vi "Ground Station to Aircraft Coms Main.vi"(11 "Instance Details":T16) -> ()   [LabVIEW 2014]
uses:
  Application Support/Stop Button/SubVI/Get Stop Button Status.vi
  MAVLink/Commands/MAV_CMD Sub VI/MAV_CMD_COMPONENT_ARM_DISARM.vi
  Telemetry/Controls/Aircraft State.ctl
  Aircraft Information/Sub VI/Get Aircraft System Status.vi
  Aircraft Information/Sub VI/Set Aircraft System Status.vi
  Aircraft Information/Sub VI/Get Aircraft Attitude.vi
  Aircraft Information/Sub VI/Get Aircraft RC.vi
  Aircraft Information/Sub VI/Get Aircraft Information.vi
  Aircraft Information/Sub VI/Get Aircraft Extra Data.vi
  Aircraft Information/Sub VI/Get Aircraft GPS.vi
  Aircraft Information/Controls/Aircraft RC Data.ctl
  Aircraft Information/Controls/Aircraft Attitude Data.ctl
  Aircraft Information/Controls/Base Mode.ctl
  Aircraft Information/Controls/Drone Information.ctl
  Aircraft Information/Controls/Aircraft Mode.ctl
  Aircraft Information/Controls/Aircraft Sensor Status Data.ctl
  GUI Design/Indicators/Status LED.ctl
  GUI Design/Indicators/Sensor Status LED CLuster.ctl
  Telemetry/Controls/Telemetry Connection Type.ctl
  SubVI/Aircraft Data Router/Controls/Known Aircraft.ctl
  SubVI/Hardware Driver/Controls/Coms Driver Interface.ctl
  MAVLink/Controls/MAVLink Optical Flow.ctl
  MAVLink/Controls/MAVLink EKF Status Report.ctl
  Aircraft Information/Controls/Aircraft Extra Data.ctl
  Aircraft Information/Controls/Aircraft GPS Data.ctl
  <vilib>/httpClient/ClientHandle.ctl
  <vilib>/httpClient/LabVIEWHTTPClient.lvlib
  Aircraft Information/Controls/GPS Fix Type.ctl
panel:
  in  "Aircraft State":T1=enum."Initialise"
  in  "Main Tab":T2(tab)
  out "Drone Information":T3={"Aircraft ID"=0, "Tag ID"="", "System Status"="", "Base Mode"={"Custom Mode"=FALSE, "Test Enabled"=FALSE, "Autonomous Mode"=FALSE, "Guided Mode"=FALSE, "Stabilization Enabled"=FALSE, "HIL Enabled"=FALSE, "Manual Mode"=FALSE, "Arm"=FALSE}, "Armed/Disarmed"=FALSE, "Battery Voltage"=0.0, "Control Mode"=enum."Stabalise", "Initialisation"=0, "Coms with aircraft good"=FALSE, "Mode"="", "Mission Uploaded"=FALSE} {"Initialisation" scale=0.0..100.0}
  out "Aircraft GPS Data Out":T6
  in  "ARM/DISARM":bool
  in  "Takeoff":bool
  in  "Altitude (m)":sgl
  out "Aircraft Att Data Out":T8
  out "System Status Out":T9 {"Communication Drop Rate (%)" scale=0.0..100.0; "Battery Remaining (%)" scale=0.0..100.0; "CPU Load (%)" scale=0.0..100.0}
  out "Status text":string
  in  "Clear Status Text":bool
  out "Extra Data Out":T12
  out "TX Queue State":i32(slide) scale=0.0..50.0
  out "RX Queue State":i32(slide) scale=0.0..50.0
  out "Waypoint Queue State":i32(slide) scale=0.0..50.0
  in  "param_id":string
  in  "Request Param":bool
  in  "Get Message":bool
  in  "Message Rate (hz)":u16=5
  in  "start_stop":bool
  in  "req_stream_id":T15(ring)
  in  "Release Control":bool
  out "Aircraft RC Data Out":T20
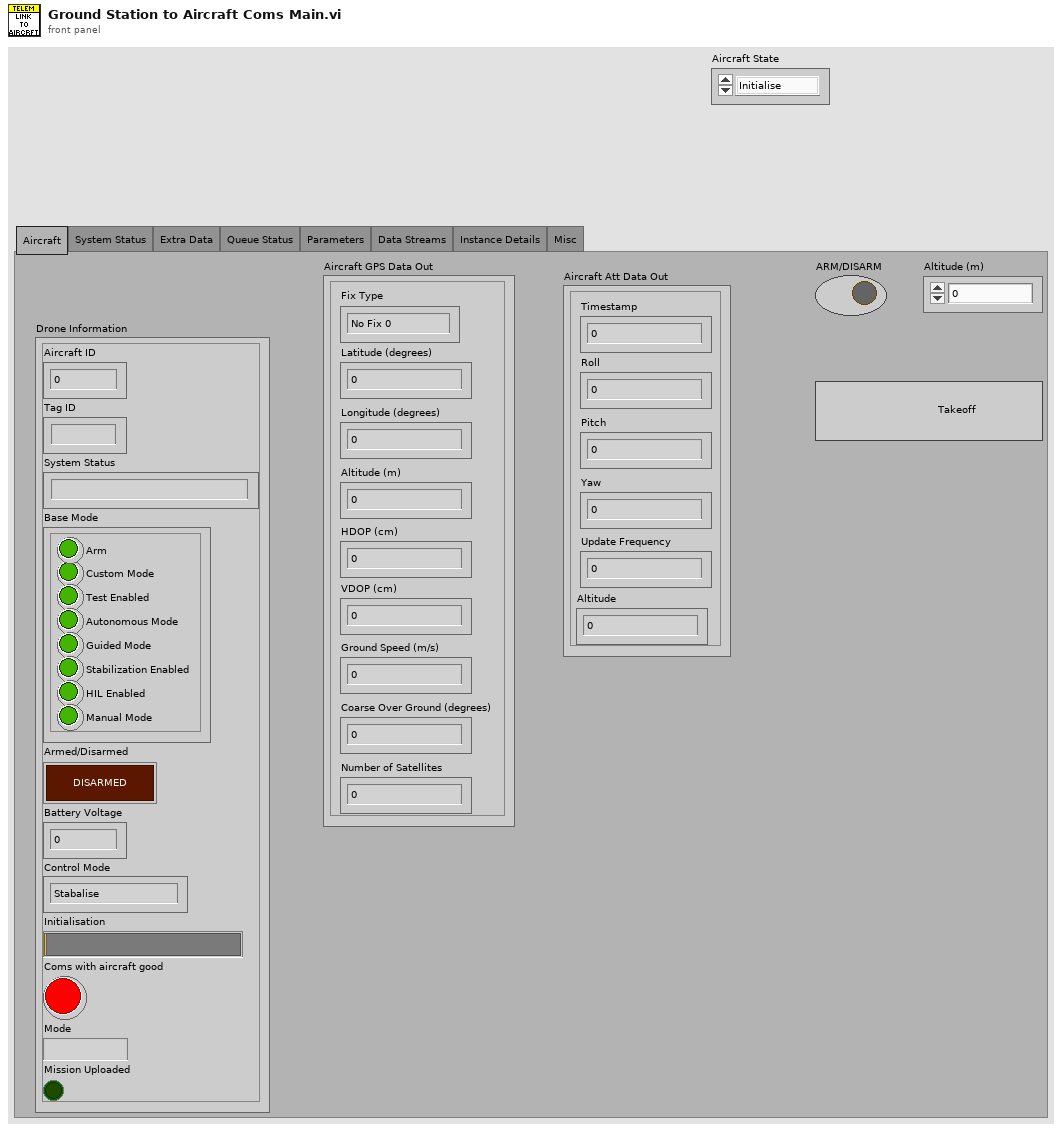
[diagram p1: front panel]
types:
  T1 = typedef "Aircraft State.ctl" = enum16{"Connected", "Initialise", "Disconnected"}
  T2 = enum32{"Aircraft", "System Status", "Extra Data", "Queue Status", "Parameters", "Data Streams", "Instance Details", "Misc"}
  T3 = typedef "Drone Information.ctl" = cluster{"Aircraft ID":u8, "Tag ID":string, "System Status":string, "Base Mode":T4, "Armed/Disarmed":bool, "Battery Voltage":dbl, "Control Mode":T5, "Initialisation":u8, "Coms with aircraft good":bool, "Mode":string, "Mission Uploaded":bool}
  T4 = typedef "Base Mode.ctl" = cluster{"Custom Mode":bool, "Test Enabled":bool, "Autonomous Mode":bool, "Guided Mode":bool, "Stabilization Enabled":bool, "HIL Enabled":bool, "Manual Mode":bool, "Arm":bool}
  T5 = typedef "Aircraft Mode.ctl" = enum16{"Loiter", "Stabalise", "Failsafe", "Emergency Stop"}
  T6 = typedef "Aircraft GPS Data.ctl" = cluster{"Latitude (degrees)":dbl, "Longitude (degrees)":dbl, "Altitude (m)":dbl, "Fix Type":T7, "HDOP (cm)":u16, "VDOP (cm)":u16, "Ground Speed (m/s)":dbl, "Coarse Over Ground (degrees)":u16, "Number of Satellites":u8}
  T7 = typedef "GPS Fix Type.ctl" = enum16{"No Fix 0", "No Fix 1", "2D Fix", "3D Fix", "DGPS", "RTK"}
  T8 = typedef "Aircraft Attitude Data.ctl" = cluster{"Roll":sgl, "Pitch":sgl, "Yaw":sgl, "Timestamp":u32, "Update Frequency":dbl, "Altitude":sgl}
  T9 = typedef "Aircraft Sensor Status Data.ctl" = cluster{"Sensor Status":T10, "CPU Load (%)":dbl, "Battery Voltage (V)":dbl, "Battery Current (A)":dbl, "Battery Remaining (%)":dbl, "Communication Drop Rate (%)":dbl, "Communication Errors (%)":dbl, "Status text":string}
  T10 = typedef "Sensor Status LED CLuster.ctl" = cluster{"3D Gyro":u32, "3D Accel":u32, "3D Mag":u32, "Abs. Pressure":u32, "Diff. Pressure":u32, "GPS":T11, "Optical Flow":u32, "Vision Position":u32, "Laser Position":u32, "External Ground Truth":u32, "Angular Rate Control":u32, "Attitude Stabilisation":u32, "Yaw Position":u32, "Z Altitude Control":u32, "XY Position Control":u32, "Motor Outputs":u32, "RC Receiver":u32, "3D Gyro 2":u32, "3D Accel 2":u32, "3D Mag 2":u32, "Geofence":u32, "AHRS":u32, "Terrain":u32}
  T11 = typedef "Status LED.ctl" = u32
  T12 = typedef "Aircraft Extra Data.ctl" = cluster{"Optical Flow":T13, "RNGFND Distance (m)":sgl, "RNGFND Voltage":sgl, "EKF Status Report":T14}
  T13 = typedef "MAVLink Optical Flow.ctl" = cluster{"Time (usec)":u64, "Flow Comp mx":sgl, "Flow Comp my":sgl, "Ground Distance (m)":sgl, "Flow x":i16, "Flow y":i16, "Sensord ID":u8, "Quality":u8}
  T14 = typedef "MAVLink EKF Status Report.ctl" = cluster{"EKF Status Flags":cluster{"Attitude Estimate":bool, "Horizontal Velocity":bool, "Vertical Velocity":bool, "Horizontal POS Relative":bool, "Horizontal POS Absolute":bool, "Vertical POS Relative":bool, "Vertical POS Absolute":bool, "Vertical POS AGL":bool, "Contstant POS Mode":bool, "Predicted Horizontal POS Relative":bool, "Predicted Horizontal POS Absolute":bool}, "Velocity Variance":sgl, "Horizontal POS Variance":sgl, "Vertical POS Variance":sgl, "Compass Variance":sgl, "Terrain Altitude Variance":sgl}
  T15 = enum16{"ALL", "RAW_SENSORS", "EXTENDED_STATUS", "RC_CHANNELS", "RAW_CONTROLLER", "POSITION", "EXTRA1", "EXTRA2", "EXTRA3"}
  T16 = typedef "Known Aircraft.ctl" = cluster{"Aircraft ID":u8, "Aircraft Receive queue Ref":refnum<queue>, "Aircraft Transmit queue Ref":refnum<queue>, "Waypoint Queue Ref":refnum<queue>, "Connection Details":T17}
  T17 = typedef "Coms Driver Interface.ctl" = cluster{"Connection Type":T18, "UDP connection ID":refnum<k16>, "Serial COM port ID":refnum<visa-resource-name>, "IP Address of Aircraft":u32, "Remote Master Details":cluster{"Remote Master client handle":T19, "Base Path of Web Service":string}, "UDP TX Port of Aircraft":u16}
  T18 = typedef "Telemetry Connection Type.ctl" = enum16{"Serial", "UDP", "Remote Master"}
  T19 = typedef "LabVIEWHTTPClient.lvlib/ClientHandle.ctl" = refnum<k1>
  T20 = typedef "Aircraft RC Data.ctl" = cluster{"Channel 1 Min":i16, "Channel 1 Max":i16, "Channel 2 Min":i16, "Channel 2 Max":i16, "Channel 3 Min":i16, "Channel 3 Max":i16, "Channel 4 Min":i16, "Channel 4 Max":i16}
  T21 = cluster{"req_message_rate":u16, "target_system":u8, "target_component":u8, "req_stream_id":enum16{"ALL", "RAW_SENSORS", "EXTENDED_STATUS", "RC_CHANNELS", "RAW_CONTROLLER", "POSITION", "EXTRA1", "EXTRA2", "EXTRA3"}, "start_stop":bool}
  T22 = cluster{"chan1_raw":u16, "chan2_raw":u16, "chan3_raw":u16, "chan4_raw":u16, "chan5_raw":u16, "chan6_raw":u16, "chan7_raw":u16, "chan8_raw":u16, "target_system":u8, "target_component":u8}
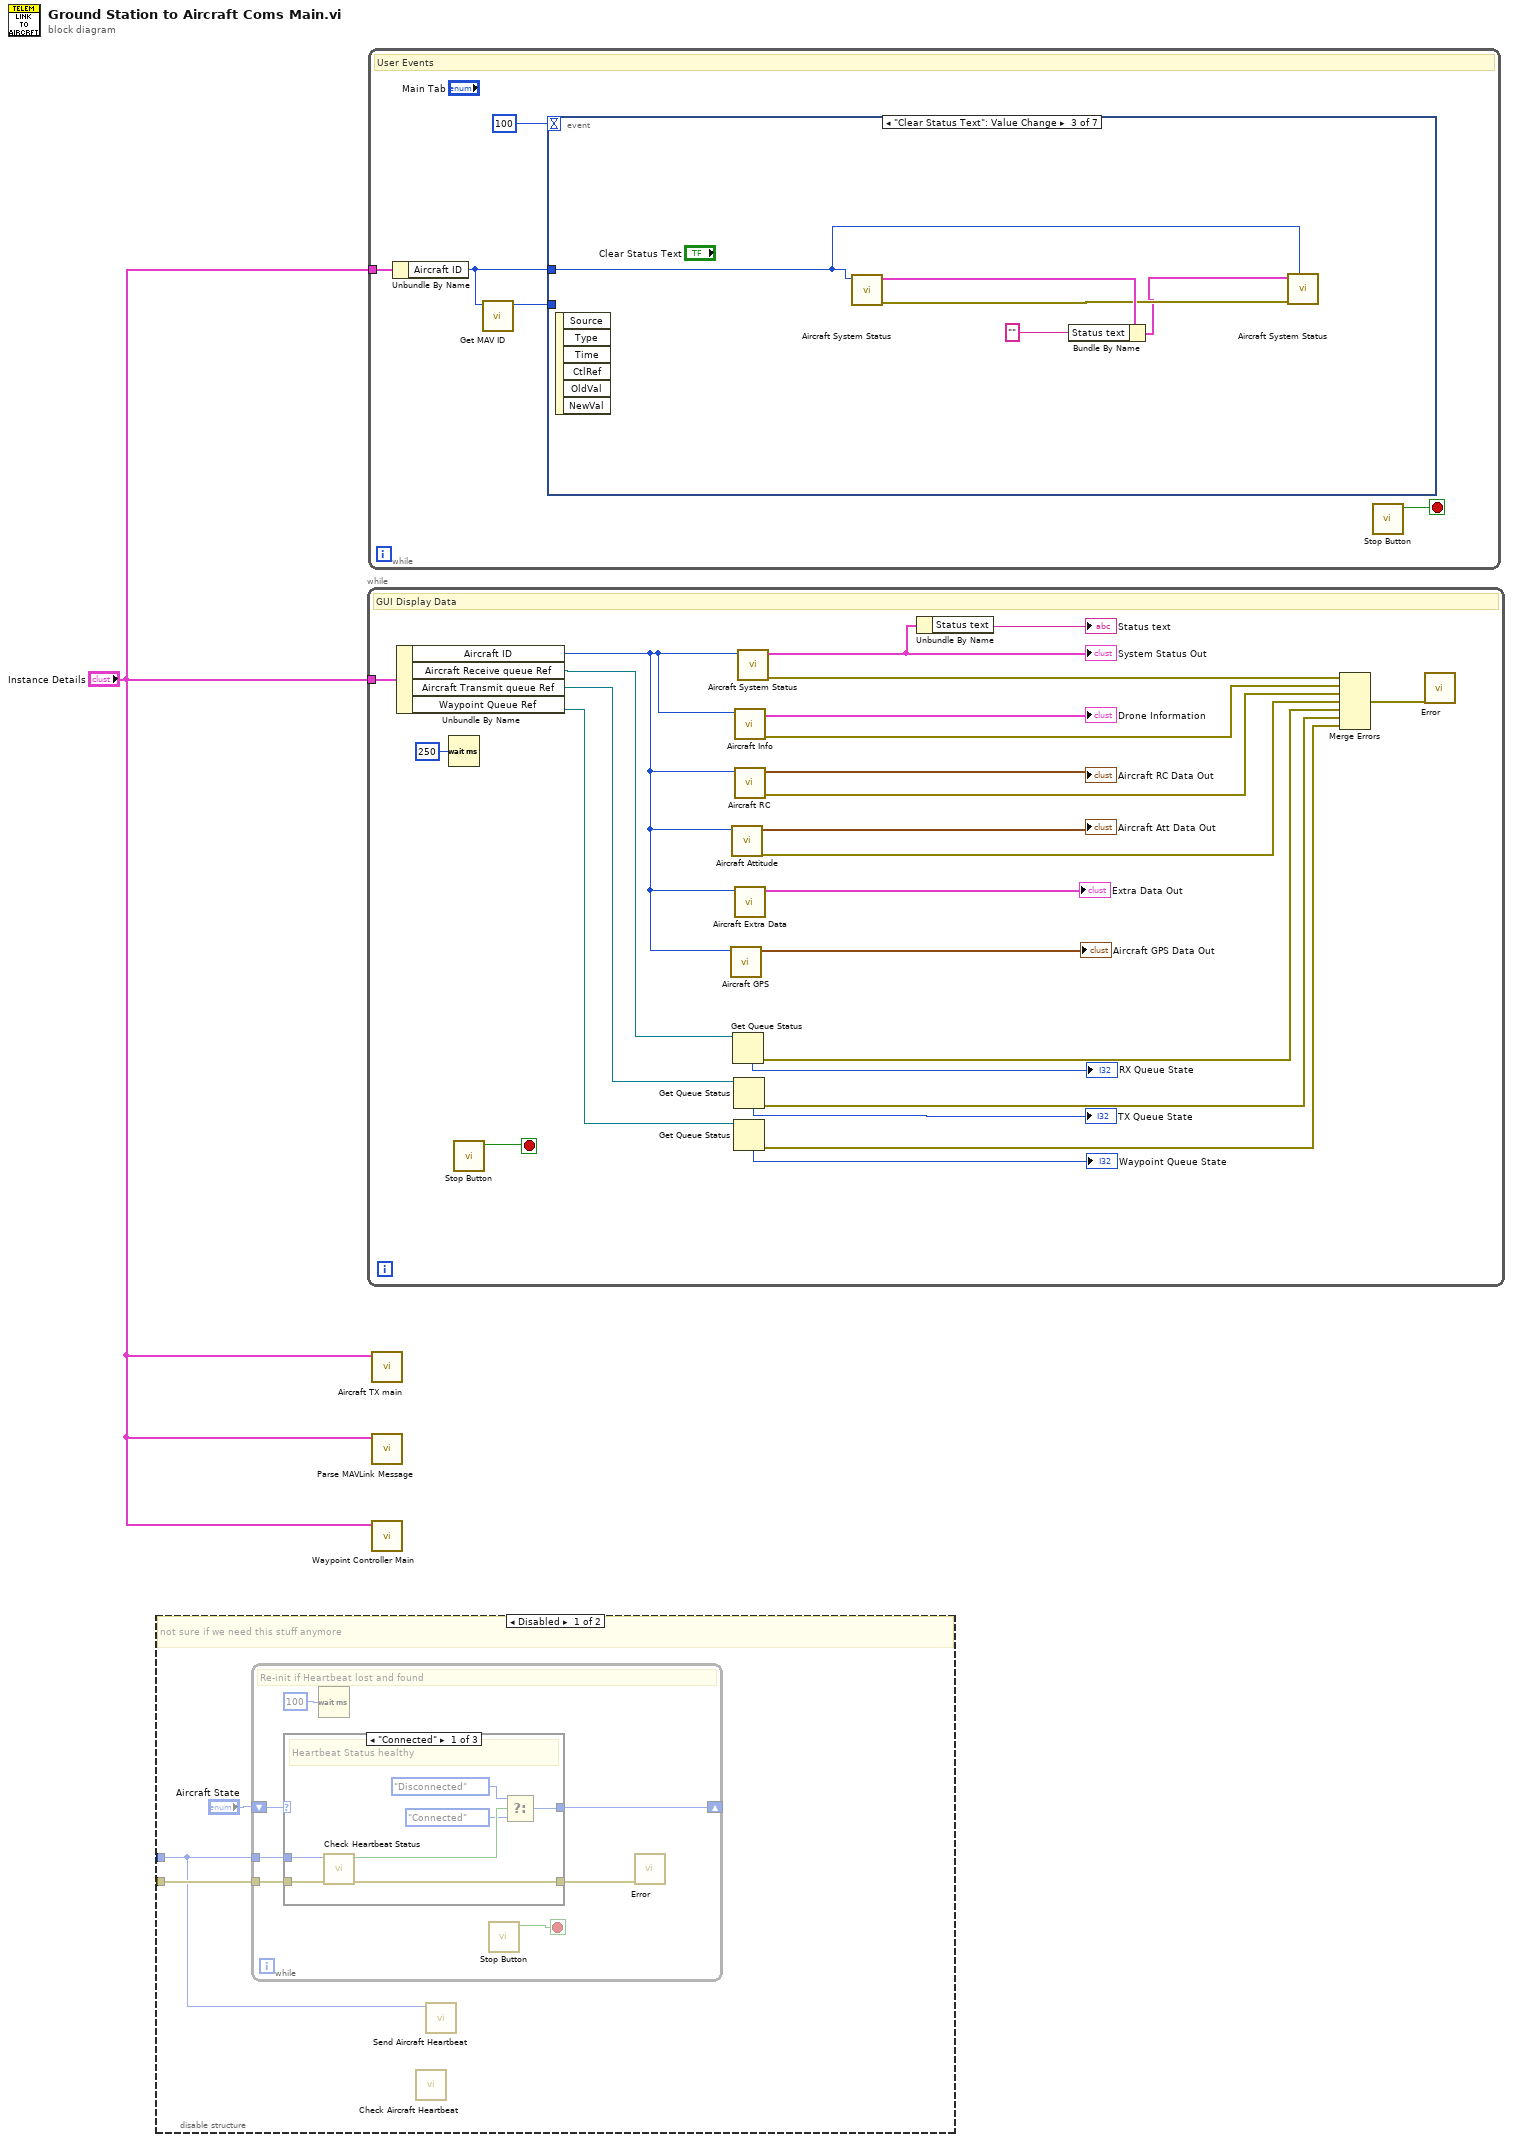
[diagram p0: block diagram]
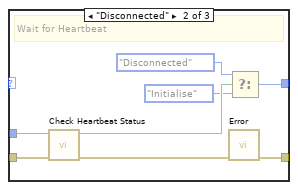
[diagram p2: hidden frame]
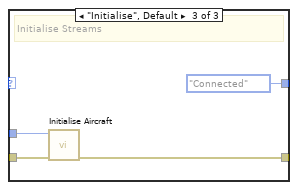
[diagram p3: hidden frame]
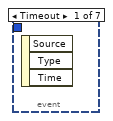
[diagram p5: hidden frame]
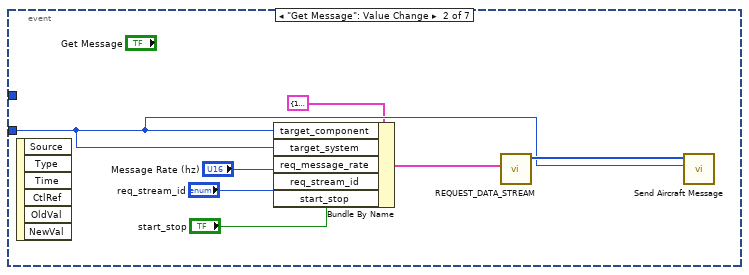
[diagram p6: hidden frame]
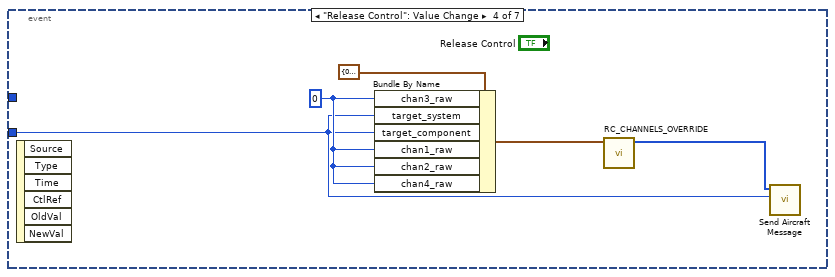
[diagram p7: hidden frame]
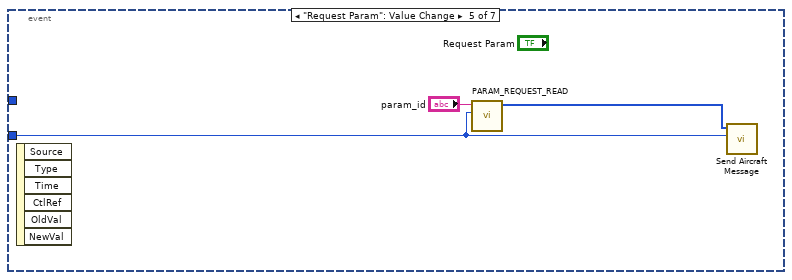
[diagram p8: hidden frame]
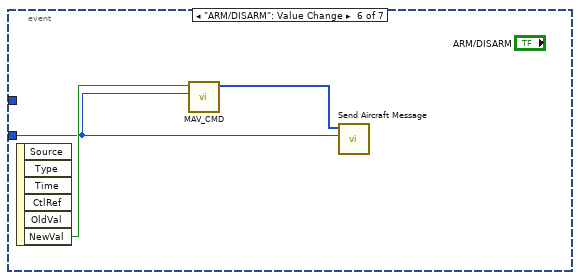
[diagram p9: hidden frame]
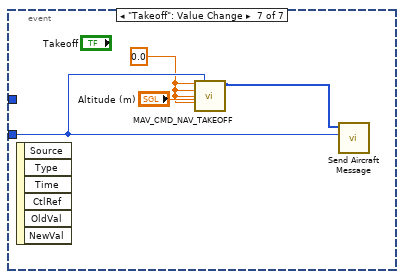
[diagram p10: hidden frame]
diagram:
  n1 = disable-structure shown="Disabled" {
    disable-tunnel: _ -> [w2 _]
    disable-tunnel: _ -> [w3 _]
    frame Disabled {
      # "not sure if we need this stuff anymore"
      n2 = while {
        tunnel: w3 -> [w7]
        tunnel: w2 -> [w11]
        shift-right: [w8] -> _
        shift-left: "Aircraft State" -> [w9]
        stop <- w10 stop-if-true
        # "Re-init if Heartbeat lost and found"
        n3 = case shown="\"Connected\"" w9 {
          tunnel: w7 -> [w18 w25 w29]
          tunnel: w11 -> [w17 w24 w28]
          tunnel: [w12 w20 Aircraft_State."Connected" ("Aircraft State")] -> w8
          tunnel: [w13 w19 w27] -> w5
          frame "Connected" {
            # "Heartbeat Status healthy"
            n4 = call "Check Heartbeat Status.vi"("Error In"=w18, "Aircraft ID"=w17) -> ("Error Out"=w13:errorcluster, "Heartbeat Lost"=w16:bool)  [unwired: 8 in]
            n5 = Select(t=Aircraft_State."Disconnected" ("Aircraft State"), s=w16, f=Aircraft_State."Connected") -> (s? t:f=w12:T1)
          }
          frame "Disconnected" {
            # "Wait for Heartbeat"
            n6 = call "Check Heartbeat Status.vi"("Error In"=w25, "Aircraft ID"=w24) -> ("Error Out"=w23:errorcluster, "Heartbeat Lost"=w26:bool)  [unwired: 8 in]
            n7 = call "Error.vi"("Error In"=w23) -> ("Error Out"=w19:errorcluster)  [unwired: 10 in]
            n8 = Select(t=Aircraft_State."Disconnected", s=w26, f=Aircraft_State."Initialise" ("Aircraft State")) -> (s? t:f=w20:T1)
          }
          frame "Initialise", Default {
            # "Initialise Streams"
            n9 = call "Initialise Aircraft.vi"("error IO"=w29, "Aircraft ID"=w28) -> ("error out"=w27:errorcluster)  [unwired: 9 in]
          }
        }
        n10 = Wait (ms)(milliseconds to wait=u32 100) -> ()  [unwired: 1 out]
        n11 = call-poly "Stop Button.vi"() -> ("Stop ButtonOut"=w10:bool)  [unwired: 10 in, 1 out]
        n12 = call "Error.vi"("Error In"=w5) -> ()  [unwired: 10 in, 1 out]
      }
      n13 = call "Check Aircraft Heartbeat.vi"() -> ()  [unwired: 11 in, 1 out]
      n14 = call "Send Aircraft Heartbeat.vi"("Aircraft ID"=w2) -> ()  [unwired: 11 in]
    }
    frame Enabled {
    }
  }
  n15 = while {
    tunnel: "Instance Details" -> [w53]
    stop <- w55 stop-if-true
    # "GUI Display Data"
    n16 = Unbundle By Name(w53) -> ("Aircraft ID"=w31:u8, "Aircraft Receive queue Ref"=w52:refnum<queue>, "Aircraft Transmit queue Ref"=w51:refnum<queue>, "Waypoint Queue Ref"=w50:refnum<queue>)
    n17 = Wait (ms)(milliseconds to wait=u32 250) -> ()  [unwired: 1 out]
    n18 = call-poly "Stop Button.vi"() -> ("Stop ButtonOut"=w55:bool)  [unwired: 10 in, 1 out]
    n19 = call-poly "Aircraft GPS.vi"("Aircraft ID"=w31) -> ("Aircraft GPS Data Out"=→"Aircraft GPS Data Out":T6)  [unwired: 9 in, 1 out]
    n20 = call-poly "Aircraft Attitude.vi"("Aircraft ID"=w31) -> ("Error Out"=w38:errorcluster, "Aircraft Att Data Out"=→"Aircraft Att Data Out":T8)  [unwired: 9 in]
    n21 = Get Queue Status(queue=w52) -> (error out=w37:errorcluster, # elements in queue=→"RX Queue State":i32)  [unwired: 2 in, 6 out]
    n22 = Get Queue Status(queue=w51) -> (error out=w36:errorcluster, # elements in queue=→"TX Queue State":i32)  [unwired: 2 in, 6 out]
    n23 = Get Queue Status(queue=w50) -> (error out=w35:errorcluster, # elements in queue=→"Waypoint Queue State":i32)  [unwired: 2 in, 6 out]
    n24 = call-poly "Aircraft Info.vi"("Aircraft ID"=w31) -> ("Error Out"=w40:errorcluster, "Aircraft Information Out"=→"Drone Information":T3)  [unwired: 9 in]
    n25 = call-poly "Aircraft RC.vi"("Aircraft ID"=w31) -> ("Error Out"=w39:errorcluster, "Aircraft RC Data"=→"Aircraft RC Data Out":T20)  [unwired: 9 in]
    n26 = call-poly "Aircraft Extra Data.vi"("Aircraft ID"=w31) -> ("Extra Data Out"=→"Extra Data Out":T12)  [unwired: 9 in, 1 out]
    n27 = call-poly "Aircraft System Status.vi"("Aircraft ID"=w31) -> ("Error Out"=w41:errorcluster, "System Status Out"=w46:T9)  [unwired: 9 in]
    "System Status Out" <- w46
    n28 = Unbundle By Name(w46) -> ("Status text"=→"Status text":string)
    n29 = Merge Errors(w41, w40, w39, w38, w37, w36, w35) -> (w34:errorcluster)
    n30 = call "Error.vi"("Error In"=w34) -> ()  [unwired: 10 in, 1 out]
  }
  n31 = while {
    tunnel: "Instance Details" -> [w57]
    stop <- w59 stop-if-true
    # "User Events"
    n32 = Unbundle By Name(w57) -> ("Aircraft ID"=w56:u8)
    n33 = call "Get MAV ID.vi"("Aircraft Index"=w56) -> ("Aircraft ID"=w58:u8)  [unwired: 9 in, 1 out]
    n34 = event shown="[2] \"Clear Status Text\": Value Change" {
      selector: _ -> [_ _ _ _ _ _ _]
      dyn-events: _ -> [_ _ _ _ _ _ _]
      timeout: 100 -> [_ _ _ _ _ _ _]
      tunnel: w58 -> [_ w65 _ w73 w78 w81 w86]
      tunnel: w56 -> [_ _ w69 _ _ _ _]
      event Timeout {
        n35 = event-data() -> ()  [unwired: 1 in, 3 out]
      }
      event "Get Message": Value Change {
        n36 = event-data() -> ()  [unwired: 1 in, 6 out]
        n37 = Bundle By Name(cluster=T21 {"req_message_rate"=10, "target_system"=0, "target_component"=0, "req_stream_id"=enum."ALL", "start_stop"=FALSE} ("Payload"), "target_component"=w65, "target_system"=w65, "req_message_rate"="Message Rate (hz)", "req_stream_id"="req_stream_id", "start_stop"="start_stop") -> (w61:T21)
        n38 = call "REQUEST_DATA_STREAM.vi"("Payload"=w61) -> ("MAVLink MSG"=w67:u8[])  [unwired: 10 in]
        n39 = call "Send Aircraft Message.vi"("Aircraft ID"=w65, "MAVLink Message"=w67) -> ()  [unwired: 9 in, 1 out]
      }
      event "Clear Status Text": Value Change {
        n40 = event-data() -> ()  [unwired: 1 in, 6 out]
        n41 = call-poly "Aircraft System Status.vi"("Aircraft ID"=w69) -> ("Error Out"=w70:errorcluster, "System Status Out"=w72:T9)  [unwired: 9 in]
        n42 = Bundle By Name(cluster=w72, "Status text"="") -> (w68:T9)
        n43 = call-poly "Aircraft System Status.vi"("Aircraft ID"=w69, "Error In"=w70, "System Status In"=w68) -> ()  [unwired: 7 in, 2 out]
      }
      event "Release Control": Value Change {
        w75 = u16 0 ("chan3_raw")
        n44 = event-data() -> ()  [unwired: 1 in, 6 out]
        n45 = Bundle By Name(cluster=T22 {"chan1_raw"=0, "chan2_raw"=0, "chan3_raw"=0, "chan4_raw"=0, "chan5_raw"=0, "chan6_raw"=0, "chan7_raw"=0, "chan8_raw"=0, "target_system"=0, "target_component"=0} ("Payload"), "chan3_raw"=w75, "target_system"=w73, "target_component"=w73, "chan1_raw"=w75, "chan2_raw"=w75, "chan4_raw"=w75) -> (w77:T22)
        n46 = call "RC_CHANNELS_OVERRIDE.vi"("Payload"=w77) -> ("MAVLink Message"=w74:u8[])  [unwired: 10 in]
        n47 = call "Send Aircraft Message.vi"("Aircraft ID"=w73, "MAVLink Message"=w74) -> ()  [unwired: 9 in, 1 out]
      }
      event "Request Param": Value Change {
        n48 = event-data() -> ()  [unwired: 1 in, 6 out]
        n49 = call "PARAM_REQUEST_READ.vi"("Target System and Target Component"=w78, "param_id"="param_id") -> ("MAVLink Message"=w79:u8[])  [unwired: 9 in]
        n50 = call "Send Aircraft Message.vi"("Aircraft ID"=w78, "MAVLink Message"=w79) -> ()  [unwired: 9 in, 1 out]
      }
      event "ARM/DISARM": Value Change {
        n51 = event-data() -> ("NewVal"=w83:bool)  [unwired: 1 in, 5 out]
        n52 = call-poly "MAV_CMD.vi"("Target System and Target Component"=w81, "ARM(T)/DISARM(F)"=w83) -> ("MAVLink Message"=w82:u8[])  [unwired: 9 in]
        n53 = call "Send Aircraft Message.vi"("Aircraft ID"=w81, "MAVLink Message"=w82) -> ()  [unwired: 9 in, 1 out]
      }
      event "Takeoff": Value Change {
        w84 = sgl 0.0 ("Yaw Angle")
        n54 = event-data() -> ()  [unwired: 1 in, 6 out]
        n55 = call "MAV_CMD_NAV_TAKEOFF.vi"("Minimum Pitch"=w84, "Aircraft ID"=w86, "Yaw Angle"=w84, "Latitude"=w84, "Longitude"=w84, "Altitude (m)"="Altitude (m)") -> ("MAVLink Message"=w87:u8[])  [unwired: 9 in]
        n56 = call "Send Aircraft Message.vi"("Aircraft ID"=w86, "MAVLink Message"=w87) -> ()  [unwired: 9 in, 1 out]
      }
    }
    n57 = call-poly "Stop Button.vi"() -> ("Stop ButtonOut"=w59:bool)  [unwired: 10 in, 1 out]
  }
  n58 = call "Aircraft TX main.vi"("Instance Details"="Instance Details") -> ()  [unwired: 11 in]
  n59 = call "Parse MAVLink Message.vi"("Instance Details"="Instance Details") -> ()  [unwired: 11 in]
  n60 = call "Waypoint Controller Main.vi"("Instance Details"="Instance Details") -> ()  [unwired: 11 in]
